vi "Calculate Measure Period.vi"(0 "Ramp Configurations":T1, 5 "Transient Response":T2[](array[typedef]) items=["Slow", "Normal", "Fast"], 11 "error in (no error)":errorcluster) -> (4 "Compliance Skip Duration":dbl[](array[numeric]), 6 "Measure Period":dbl, 8 "Compliance Check Duration":dbl, 15 "error out":errorcluster)   [LabVIEW 2024, in "devicePowerSequencerCoreLogic.lvlib"]
uses:
  devicePowerSequencerCoreLogic.lvlib
  controls/Transient Response.ctl
  controls/Ramp Configurations.ctl
  Device Power Sequencer.lvlib
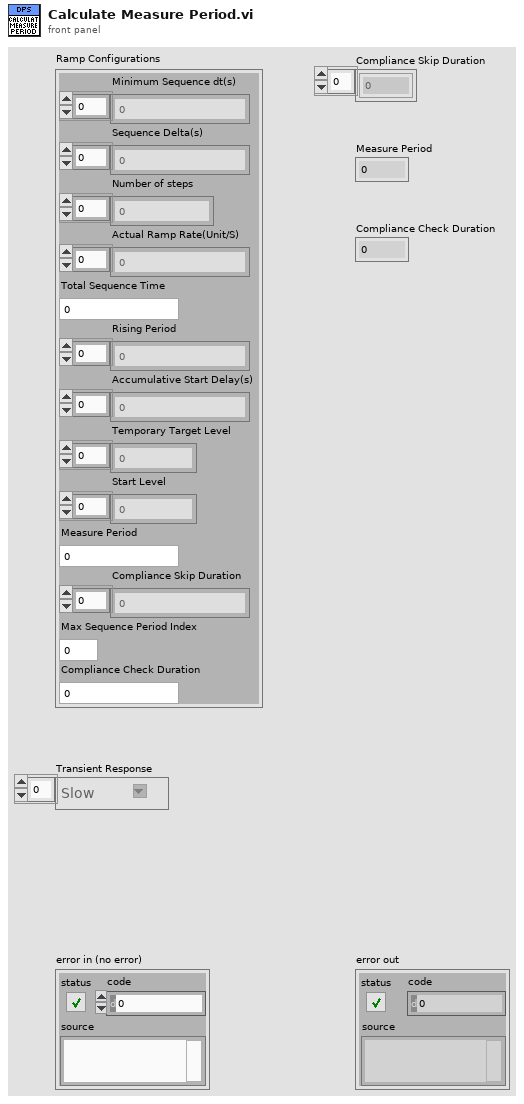
[diagram p1: front panel]
types:
  T1 = typedef "devicePowerSequencerCoreLogic.lvlib/Ramp Configurations.ctl" = cluster{"Minimum Sequence dt(s)":dbl[], "Sequence Delta(s)":dbl[], "Number of steps":i32[], "Actual Ramp Rate(Unit/S)":dbl[], "Total Sequence Time":dbl, "Rising Period":dbl[], "Accumulative Start Delay(s)":dbl[], "Temporary Target Level":dbl[], "Start Level":dbl[], "Measure Period":dbl, "Compliance Skip Duration":dbl[], "Max Sequence Period Index":i32, "Compliance Check Duration":dbl}
  T2 = typedef "Device Power Sequencer.lvlib/Transient Response.ctl" = i32
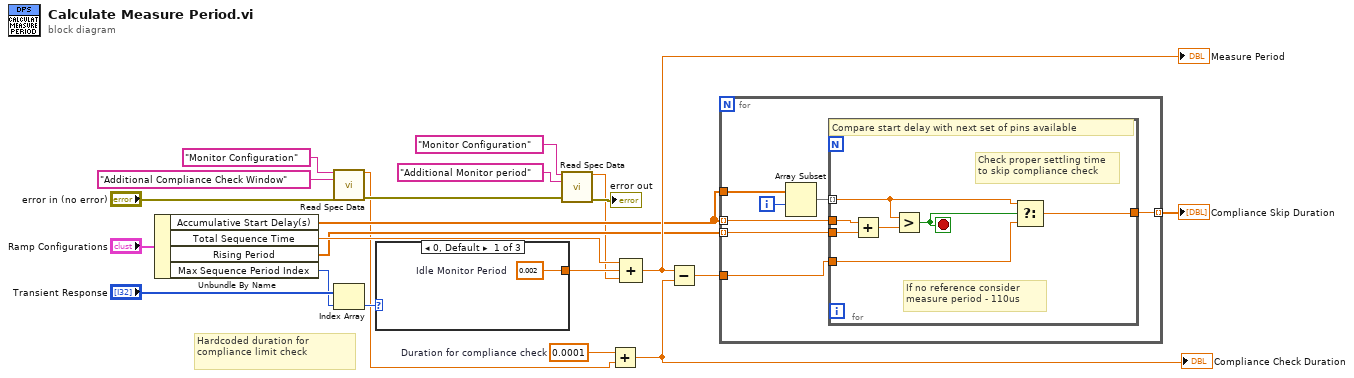
[diagram p0: block diagram]
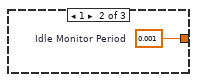
[diagram p2: hidden frame]
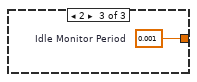
[diagram p3: hidden frame]
diagram:
  w3 = 0.0001  # Duration for compliance check
  # "Hardcoded duration for compliance limit check"
  n1 = Unbundle By Name("Ramp Configurations") -> ("Accumulative Start Delay(s)"=w15:dbl[], "Total Sequence Time"=w14:dbl, "Rising Period"=w13:dbl[], "Max Sequence Period Index"=w12:i32)
  n2 = call "Read Spec Data.vi"("section"="Monitor Configuration", "key"="Additional Compliance Check Window", "error in (no error)"="error in (no error)") -> ("value"=w2:dbl, "error out"=w4:errorcluster)  [unwired: 11 in]
  n3 = Index Array(array="Transient Response", index=w12) -> (element=w19:T2)
  n4 = case shown="0, Default" w19 {
    tunnel: [w23 w24 w25] -> w20
    frame 0, Default {
      w23 = 0.002  # Idle Monitor Period
    }
    frame 1 {
      w24 = 0.001  # Idle Monitor Period
    }
    frame 2 {
      w25 = 0.001  # Idle Monitor Period
    }
  }
  n5 = call "Read Spec Data.vi"("section"="Monitor Configuration", "key"="Additional Monitor period", "error in (no error)"=w4) -> ("value"=w10:dbl, "error out"=→"error out":errorcluster)  [unwired: 11 in]
  n6 = Add(x=w3, y=w2) -> (x+y=w1:dbl)
  "Compliance Check Duration" <- w1
  n7 = Compound Arithmetic op=ADD(w14, w20, w10) -> (w21:dbl)
  "Measure Period" <- w21
  n8 = Subtract(x=w21, y=w1) -> (x-y=w22:dbl)
  n9 = for {
    tunnel: w15 -> [w30] mode=indexing
    tunnel: w15 -> [w32]
    tunnel: [w28] -> w17 mode=indexing
    tunnel: w13 -> [w27] mode=indexing
    tunnel: w22 -> [w26]
    i -> [w31]
    n10 = Array Subset(array=w32, index=w31) -> (w29:dbl[])  [unwired: 1 in]
    n11 = for {
      tunnel: w30 -> [w36]
      tunnel: w29 -> [w38] mode=indexing
      tunnel: [w37] -> w28
      tunnel: w27 -> [w35]
      tunnel: w26 -> [w33]
      stop <- w39 stop-if-true
      # "Check proper settling time\nto skip compliance check"
      # "If no reference consider measure period - 110us"
      # "Compare start delay with next set of pins available"
      n12 = Add(x=w36, y=w35) -> (x+y=w34:dbl)
      n13 = Greater?(x=w38, y=w34) -> (0:w39:bool)
      n14 = Select(t=w38, s=w39, f=w33) -> (s? t:f=w37:dbl)
    }
  }
  "Compliance Skip Duration" <- w17
